vi "Odometer.vi"() -> ()   [LabVIEW 2014]
uses:
  <vilib>/Utility/config.llb/Write Key (Double).vi
  <vilib>/Utility/config.llb/Read Key (Double).vi
  <vilib>/Utility/config.llb/NI_LVConfig.lvlib
panel:
  in  "Close":bool
  out "Insgesamt":dbl
  in  "Maximal":dbl
  in  "Reset":bool
  in  "Pfad":path
  in  "Save":bool
  out "Drehspulinstrument":dbl(knob) scale=0.0..5500.0 scale format="%#_5g"
  in  "Aktuell":dbl
  # "Zurückgelegter Weg nach Reset"
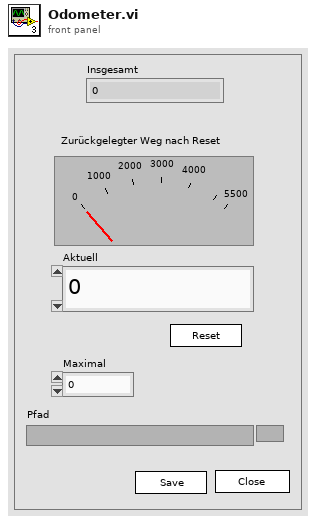
[diagram p1: front panel]
types:
  T1 = typedef "NI_LVConfig.lvlib/Config Data RefNum.ctl" = refnum<k1>
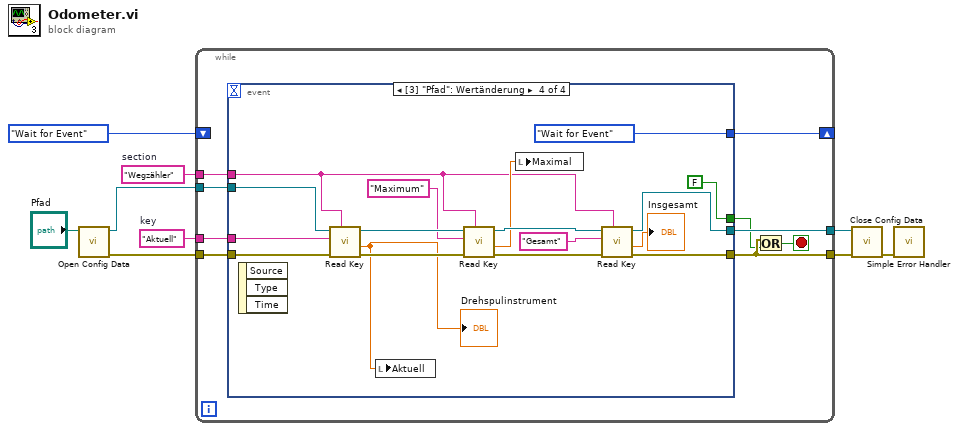
[diagram p0: block diagram]
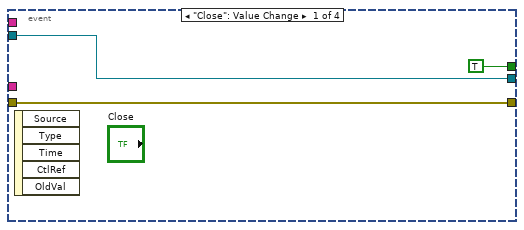
[diagram p2: hidden frame]
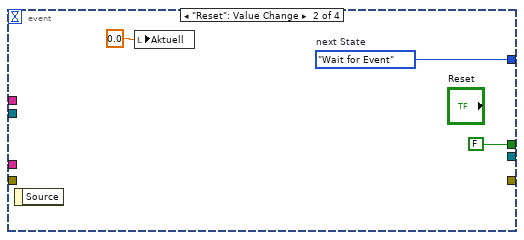
[diagram p3: hidden frame]
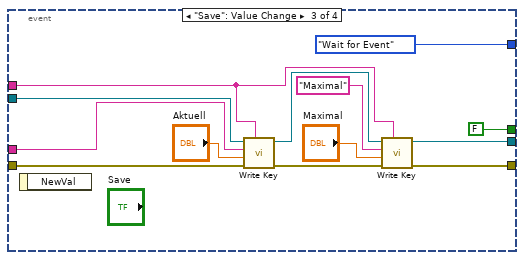
[diagram p4: hidden frame]
diagram:
  w4 = "Aktuell"  # key
  w5 = "Wegzähler"  # section
  n1 = call <vilib>:"Open Config Data.vi"("configuration file path"="Pfad") -> ("error out"=w6:errorcluster, "refnum"=w7:T1)  [unwired: 8 in, 1 out]
  n2 = while {
    shift-right: [w18] -> _
    shift-left: enum16{"Wait for Event", "Read"}."Wait for Event" -> [_]
    tunnel: w7 -> [w17]
    tunnel: w6 -> [w16]
    tunnel: w5 -> [w15]
    tunnel: w4 -> [w14]
    tunnel: [w13] -> w3
    tunnel: [w11] -> w2
    stop <- w12 stop-if-true
    n3 = event shown="[3] \"Pfad\": Wertänderung" {
      selector: _ -> [_ _ _ _]
      dyn-events: _ -> [_ _ _ _]
      timeout: _ -> [_ _ _ _]
      tunnel: w15 -> [_ _ w30 w44]
      tunnel: w14 -> [_ _ w37 w45]
      tunnel: w16 -> [w19 _ w36 w47]
      tunnel: w17 -> [w20 _ w35 w46]
      tunnel: [w20 _ w28 w42] -> w13
      tunnel: [w19 _ w27 w43] -> w11
      tunnel: [_ w22 enum16{"Wait for Event", "Read"}."Wait for Event" enum16{"Wait for Event", "Read"}."Wait for Event"] -> w18
      tunnel: [TRUE FALSE FALSE FALSE] -> w10
      event "Close": Value Change {
        n4 = event-data() -> ()  [unwired: 1 in, 5 out]
      }
      event "Reset": Value Change {
        w22 = enum16{"Wait for Event", "Read"}."Wait for Event"  # next State
        n5 = event-data() -> ()  [unwired: 1 in, 1 out]
        n6 = local write "Aktuell"(0.0 ("Numerisch")) -> ()
      }
      event "Save": Value Change {
        n7 = event-data() -> ()  [unwired: 1 in, 1 out]
        n8 = call-poly <vilib>:"Write Key.vi"("section"=w30, "error in (no error)"=w36, "value"="Aktuell", "key"=w37, "refnum"=w35) -> ("error out"=w26:errorcluster, "refnum out"=w31:T1)  [unwired: 4 in, 1 out]
        n9 = call-poly <vilib>:"Write Key.vi"("section"=w30, "error in (no error)"=w26, "value"="Maximal", "key"="Maximal", "refnum"=w31) -> ("error out"=w27:errorcluster, "refnum out"=w28:T1)  [unwired: 4 in, 1 out]
      }
      event "Pfad": Value Change {
        n10 = event-data() -> ()  [unwired: 1 in, 3 out]
        n11 = call-poly <vilib>:"Read Key.vi"("section"=w44, "error in (no error)"=w47, "key"=w45, "refnum"=w46) -> ("error out"=w53:errorcluster, "value"=w38:dbl, "refnum out"=w54:T1)  [unwired: 4 in, 1 out]
        "Drehspulinstrument" <- w38
        n12 = local write "Aktuell"(w38) -> ()
        n13 = call-poly <vilib>:"Read Key.vi"("section"=w44, "error in (no error)"=w53, "key"="Maximum", "refnum"=w54) -> ("error out"=w49:errorcluster, "value"=w48:dbl, "refnum out"=w50:T1)  [unwired: 4 in, 1 out]
        n14 = local write "Maximal"(w48) -> ()
        n15 = call-poly <vilib>:"Read Key.vi"("section"=w44, "error in (no error)"=w49, "key"="Gesamt", "refnum"=w50) -> ("error out"=w43:errorcluster, "value"=→"Insgesamt":dbl, "refnum out"=w42:T1)  [unwired: 4 in, 1 out]
      }
    }
    n16 = Or(x=w11, y=w10) -> (x .or. y?=w12:bool)
  }
  n17 = call <vilib>:"Close Config Data.vi"("error in (no error)"=w2, "refnum"=w3) -> ("error out"=w1:errorcluster)  [unwired: 8 in, 1 out]
  n18 = call <vilib>:"Simple Error Handler.vi"("error in (no error)"=w1) -> ()  [unwired: 4 in, 5 out]
